vi "LVClass_Pupil Get Nb Enlighted Subapertures.vi"(0 "Pupil in":refnum<class "Pupil.lvclass">, 11 "error in (no error)":errorcluster) -> (4 "Pupil out":refnum<class "Pupil.lvclass">, 6 "nb_enlighted_subapertures":i32, 15 "error out":errorcluster)   [LabVIEW 2020, in "Pupil.lvclass"]
doc: "Get Pupil buffer.\n\n--------------------------------------------------------------------------------\n\n<B>PupilIn </B> : Pupil object.\n<B>PupilOut </B> : Pupil object.\n<B>data </B> : Pupil buffer.\n<B>ErrorIn </B> : Error\n<B>ErrorOut </B> : Error\n\n--------------------------------------------------------------------------------"
uses:
  Pupil.lvclass
  Pupil.lvclass/Pupil.ctl
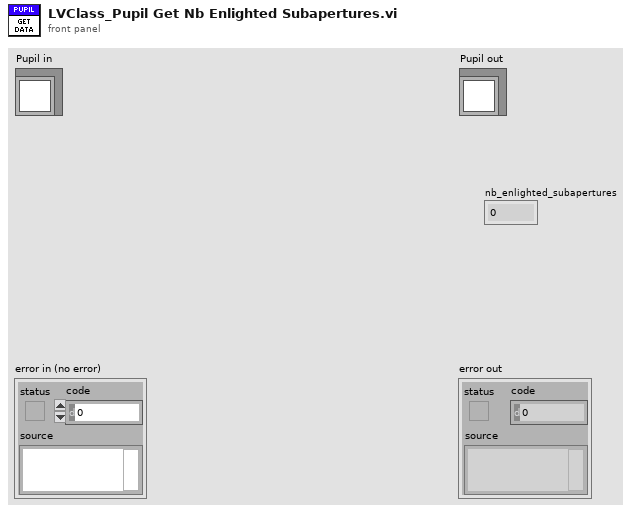
[diagram p1: front panel]
types:
  T1 = typedef "ClassID.ctl" = i64
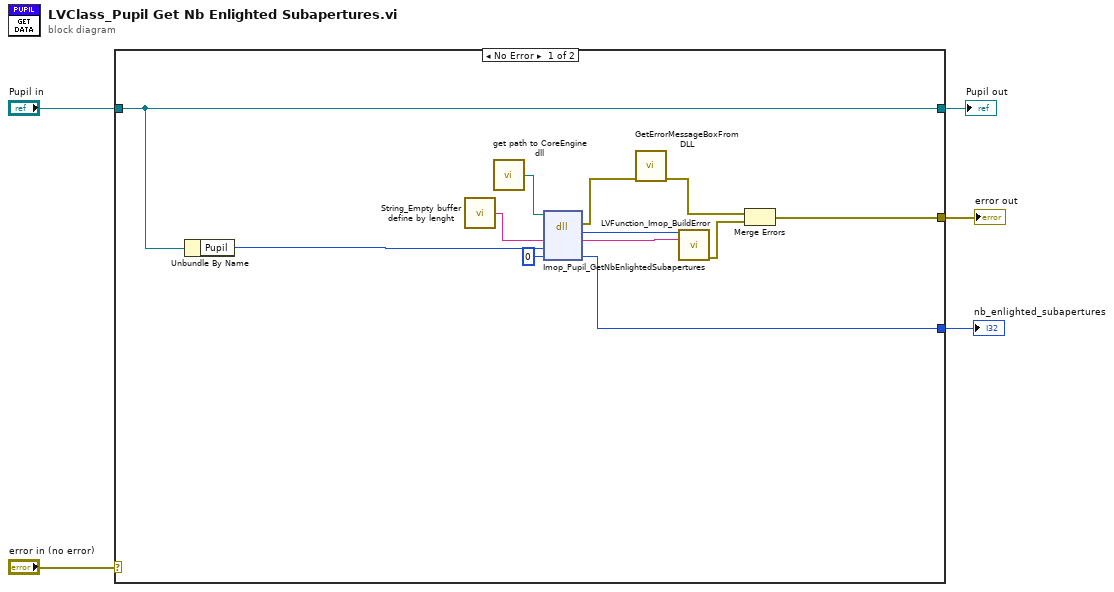
[diagram p0: block diagram]
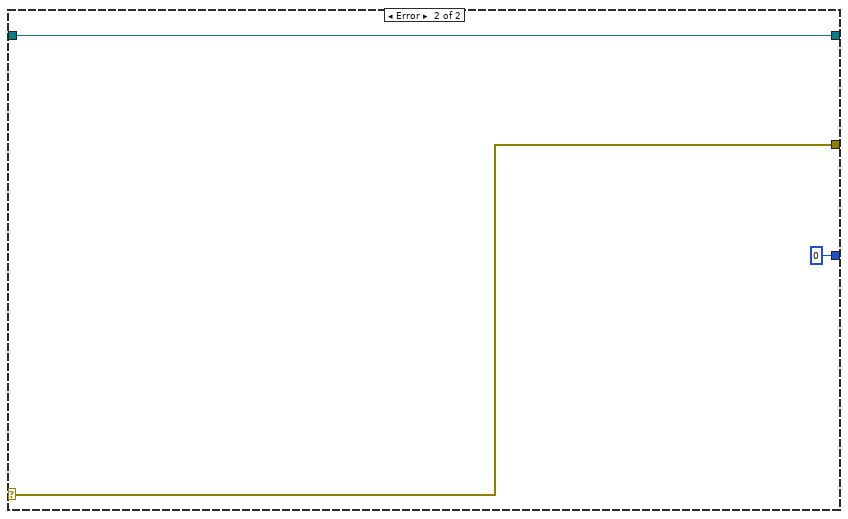
[diagram p2: hidden frame]
diagram:
  n1 = case shown="No Error" "error in (no error)" {
    selector: "error in (no error)" -> [_ w20]
    tunnel: [w9 w20] -> w5
    tunnel: [w8 w19] -> w4
    tunnel: "Pupil in" -> [w8 w19]
    tunnel: [w7 0 ("nb_enlighted_subapertures")] -> w1
    frame No Error {
      n2 = Unbundle By Name(w8) -> ("Pupil"=w12:T1)
      n3 = call "String_Empty buffer define by lenght.vi"() -> ("Empty buffer"=w17:string)  [unwired: 1 in]
      n4 = call "get path to CoreEngine dll.vi"() -> ("path to wavekit library"=w14:path)  [unwired: 14 in, 1 out]
      n5 = dll-call lib="D:/2_trunk/Soft_haso/ImOpCoreEngine4_LV2011/DLLs/ImopEngine4_vc100.dll" fn="Imop_Pupil_GetNbEnlightedSubapertures"(path in=w14, "message"=w17, "objet"=w12, "nb_enlighted_subapertures"=0) -> (error out=w13:errorcluster, "return type"=w15:i32, "message"=w16:string, "nb_enlighted_subapertures"=w7:i32)  [unwired: 3 in, 1 out]
      n6 = call "GetErrorMessageBoxFromDLL.vi"("error IN"=w13) -> ("error OUT"=w11:errorcluster)  [unwired: 10 in]
      n7 = call "LVFunction_Imop_BuildError.vi"("code"=w15, "String to Prepend to source (\"\")"=w16) -> ("error out"=w10:errorcluster)  [unwired: 13 in]
      n8 = Merge Errors(w11, w10) -> (w9:errorcluster)
    }
    frame Error {
    }
  }
  "error out" <- w5
  "Pupil out" <- w4
  "nb_enlighted_subapertures" <- w1
